vi "Actor Core.vi"(8 "error in":errorcluster, 11 "Solenoid in":refnum<class "Solenoid.lvclass">) -> (0 "error out":errorcluster, 3 "Actor out":refnum<class "Actor.lvclass">)   [LabVIEW 2018, in "Feeder Actor.lvlib" / "Solenoid.lvclass"]
doc: "The user interface for this panel.\n\n----\nPlease see the following web address for additional documentation and tutorial information:\nhttp://www.mooregoodideas.com/mgi-panel-manager/\n\nAuthor: Derek Trepanier\n\nCopyright (c) 2018, Moore Good Ideas, Inc.\n\nAll rights reserved.\n\nRedistribution and use in source and binary forms, with or without modification, are permitted provided that the following conditions are met:\n\n * Redistributions of source code must retain the above copyright notice, this list of conditions and the following disclaimer.\n * Redistributions in binary form must reproduce the above copyright notice, this list of conditions and the following disclaimer in the documentation and/or other materials provided with the distribution.\n * Neither the name of Moore Good Ideas, Inc. nor the names of its contributors may be used to endorse or promote products derived from this software without specific prior written permission.\n\nTHIS SOFTWARE IS PROVIDED BY THE COPYRIGHT HOLDERS AND CONTRIBUTORS \"AS IS\" AND ANY EXPRESS OR IMPLIED WARRANTIES, INCLUDING, BUT NOT LIMITED TO, THE IMPLIED WARRANTIES OF MERCHANTABILITY AND FITNESS FOR A PARTICULAR PURPOSE ARE DISCLAIMED. IN NO EVENT SHALL THE COPYRIGHT OWNER OR CONTRIBUTORS BE LIABLE FOR ANY DIRECT, INDIRECT, INCIDENTAL, SPECIAL, EXEMPLARY, OR CONSEQUENTIAL DAMAGES (INCLUDING, BUT NOT LIMITED TO, PROCUREMENT OF SUBSTITUTE GOODS OR SERVICES; LOSS OF USE, DATA, OR PROFITS; OR BUSINESS INTERRUPTION) HOWEVER CAUSED AND ON ANY THEORY OF LIABILITY, WHETHER IN CONTRACT, STRICT LIABILITY, OR TORT (INCLUDING NEGLIGENCE OR OTHERWISE) ARISING IN ANY WAY OUT OF THE USE OF THIS SOFTWARE, EVEN IF ADVISED OF THE POSSIBILITY OF SUCH DAMAGE."
uses:
  Solenoid.lvclass
  C:/Program Files/National Instruments/LabVIEW 2018/vi.lib/MGI/Panel Manager/Panel Actor/Panel Actor/Panel Actor.lvclass
  <vilib>/ActorFramework/Actor/Actor.lvclass
  Solenoid.lvclass/Solenoid.ctl
  <vilib>/ActorFramework/Message Enqueuer/Message Enqueuer.lvclass/Message Enqueuer.ctl
  <vilib>/ActorFramework/Message Enqueuer/Enqueue.vi
  Solenoid Messages/Switch Solenoid Msg/Switch Solenoid Msg.lvclass
  C:/Program Files/National Instruments/LabVIEW 2018/vi.lib/ActorFramework/Message/Message.lvclass
  <vilib>/ActorFramework/Message Priority Queue/Priority Enqueue.vi
  <vilib>/ActorFramework/Message Enqueuer/Message Enqueuer.lvclass
  <vilib>/MGI/Panel Manager/Panel Actor/Panel Actor/Panel Actor.lvclass
  ADM/Main.lvlib
panel:
  out "Status":bool
  in  "Aerosol":bool
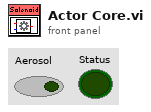
[diagram p1: front panel]
types:
  T1 = enum8{"Enabled", "Disabled", "Disabled and Grayed Out"}
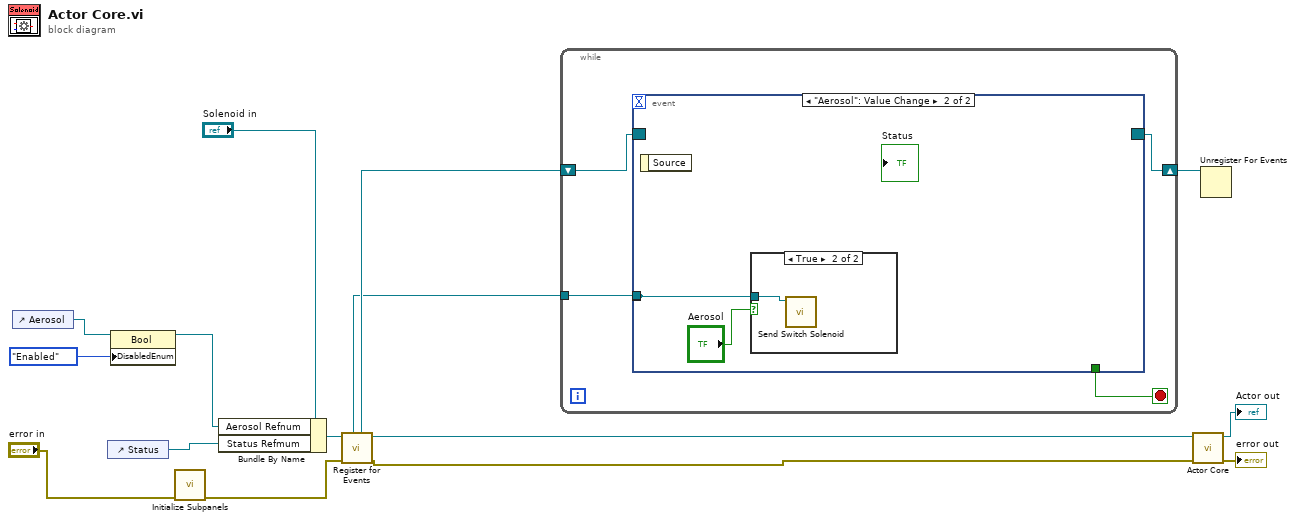
[diagram p0: block diagram]
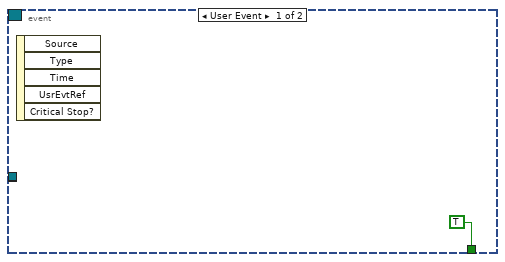
[diagram p2: hidden frame]
diagram:
  n1 = control-ref of="Aerosol"() -> (w3:refnum<vi>)
  n2 = control-ref of="Status"() -> (w5:refnum<vi>)
  n3 = property class="Bool"(reference=w3, "DisabledEnum"=T1."Enabled" ("Disabled")) -> (reference out=w2:refnum<vi>)  [unwired: 1 in, 1 out]
  n4 = call "Initialize Subpanels.vi"("error in (no error)"="error in") -> ("error out"=w9:errorcluster)  [unwired: 10 in]
  n5 = Bundle By Name(cluster="Solenoid in", "Aerosol Refnum"=w2, "Status Refmum"=w5) -> (w6:refnum<class "Solenoid.lvclass">)
  n6 = call <vilib>:"Register for Events.vi"("Error In"=w9, "Panel Actor in"=w6) -> ("Error Out"=w8:errorcluster, "Panel Actor out"=w10:refnum<class "Solenoid.lvclass">, "Pnl Actor"=w7:refnum<event-registration>, "Self Enqueuer"=w1:refnum<class "Message Enqueuer.lvclass">)  [unwired: 6 in]
  n7 = while {
    shift-right: [w17] -> w13
    shift-left: w7 -> [w19]
    tunnel: w1 -> [w16]
    stop <- w18 stop-if-true
    n8 = event shown="[1] \"Aerosol\": Value Change" {
      selector: w19 -> [_ _]
      dyn-events: [_ _] -> w17
      timeout: _ -> [_ _]
      tunnel: [TRUE _] -> w18
      tunnel: [_ w21] -> _
      tunnel: w16 -> [_ w21]
      event User Event {
        n9 = event-data() -> ()  [unwired: 1 in, 5 out]
      }
      event "Aerosol": Value Change {
        n10 = event-data() -> ()  [unwired: 1 in, 1 out]
        n11 = case shown="True" "Aerosol" {
          tunnel: w21 -> [_ w23]
          frame False {
          }
          frame True {
            n12 = call "Send Switch Solenoid.vi"("Message Enqueuer in"=w23) -> ()  [unwired: 9 in, 2 out]
          }
        }
      }
    }
  }
  n13 = call-parent "Actor Core.vi"("error in"=w8, "Panel Actor in"=w10) -> ("error out"=→"error out":errorcluster, "Actor out"=→"Actor out":refnum<class "Actor.lvclass">)  [unwired: 8 in]
  n14 = Unregister For Events(event registration refnum=w13) -> ()  [unwired: 1 in, 1 out]
